vi "Sine Wave Generator T10.vi"(8 "error in (no error)":errorcluster, 11 "IVI Refnum in":refnum<k15>) -> (0 "error out":errorcluster, 3 "pass":bool[](array[boolean]))   [LabVIEW 2021]
uses:
  <instrlib>/niDigital/niDigital.llb/niDigital Selected Function.ctl
  <instrlib>/niDigital/niDigital.llb/niDigital Burst Pattern (Pass Fail).vi
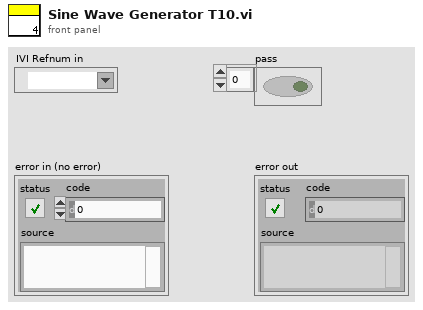
[diagram p1: front panel]
types:
  T1 = typedef "niDigital Selected Function.ctl" = i32
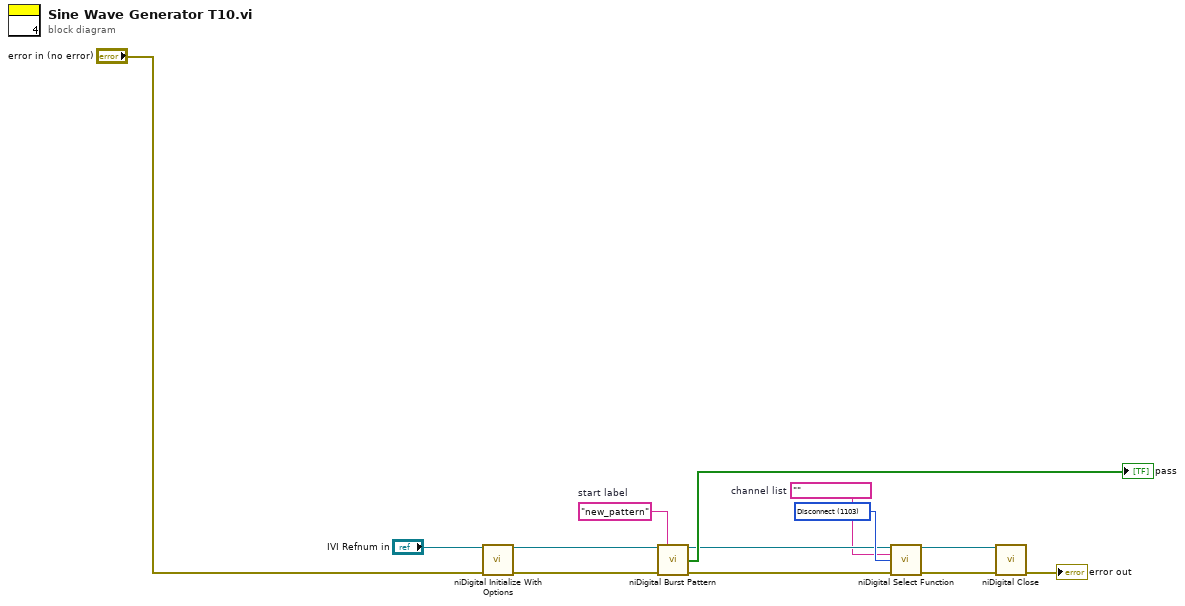
[diagram p0: block diagram]
diagram:
  w8 = T1 1103 items=["Digital"=1100, "PPMU"=1101, "Off"=1102, "Disconnect"=1103] ("function")
  w3 = ""  # channel list
  w12 = "new_pattern"  # start label
  n1 = call <instrlib>:"niDigital Initialize With Options.vi"("resource name"="IVI Refnum in", "error in"="error in (no error)") -> ("instrument handle"=w11:refnum<k15>, "error out"=w10:errorcluster)  [unwired: 12 in]
  n2 = call-poly <instrlib>:"niDigital Burst Pattern.vi"("instrument handle"=w11, "start label"=w12, "error in"=w10) -> ("instrument handle out"=w7:refnum<k15>, "pass"=→"pass":bool[], "error out"=w6:errorcluster)  [unwired: 10 in]
  n3 = call <instrlib>:"niDigital Select Function.vi"("instrument handle"=w7, "channel list"=w3, "function"=w8, "error in"=w6) -> ("instrument handle out"=w5:refnum<k15>, "error out"=w4:errorcluster)  [unwired: 10 in]
  n4 = call <instrlib>:"niDigital Close.vi"("instrument handle"=w5, "error in"=w4) -> ("error out"=→"error out":errorcluster)  [unwired: 13 in]
